vi "Project Names.vi"(8 "Error In":errorcluster, 11 "App In":refnum<vi>) -> (0 "Error Out":errorcluster, 2 "Project Names":string[](array[string]), 3 "App Out":refnum<vi>)   [LabVIEW 2017, in "Bookmark Manager.lvlib"]
uses:
  Bookmark Manager.lvlib
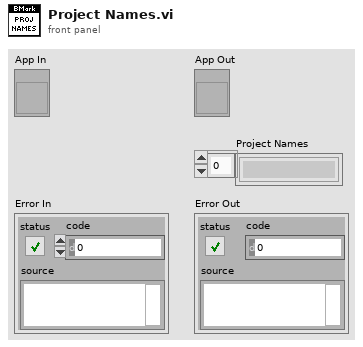
[diagram p1: front panel]
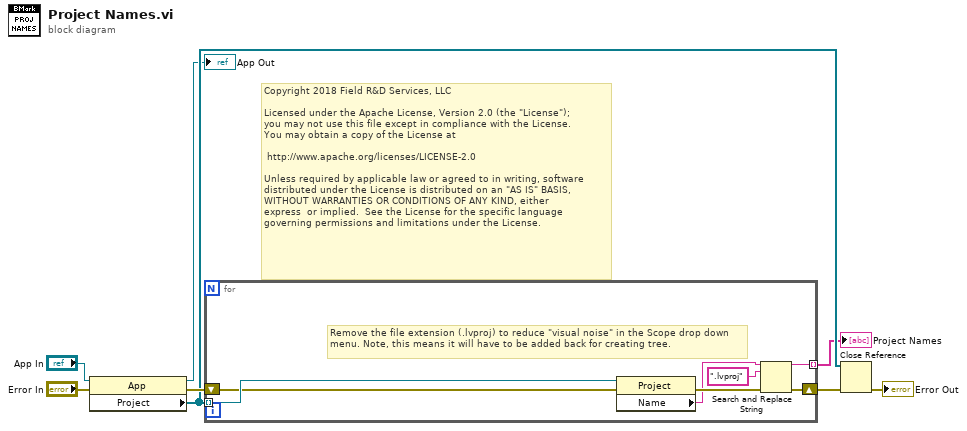
[diagram p0: block diagram]
diagram:
  # "Copyright 2018 Field R&D Services, LLC\n\nLicensed under the Apache License, Version 2.0 (the \"License\");\nyou may not use this file except in compliance with the License.\nYou may obtain a copy of the License at\n\n\thttp://www.apache.org/licenses/LICENSE-2.0\n\nUnless required by applicable law or agreed to in writing, software\ndistributed under the License is distributed on an \"AS IS\" BASIS,\nWITHOUT WARRANTIES OR CONDITIONS OF ANY KIND, either \nexpress  or implied.  See the License for the specific language \ngoverning permissions and limitations under the License."
  n1 = property class="App"(reference="App In", error in="Error In") -> (reference out=→"App Out":refnum<vi>, error out=w7:errorcluster, "Project"=w5:refnum<vi>[])
  n2 = for {
    shift-right: [w12] -> w6
    shift-left: w7 -> [w14]
    tunnel: w5 -> [w15] mode=indexing
    tunnel: [w9] -> w1 mode=indexing
    # "Remove the file extension (.lvproj) to reduce \"visual noise\" in the Scope drop down menu. Note, this means it will have to be added back for creating tree."
    n3 = property class="Project"(reference=w15, error in=w14) -> (error out=w13:errorcluster, "Name"=w11:string)  [unwired: 1 out]
    n4 = Search and Replace String(input string=w11, search string=".lvproj", error in=w13) -> (result string=w9:string, error out=w12:errorcluster)  [unwired: 5 in, 2 out]
  }
  "Project Names" <- w1
  n5 = Close Reference(reference=w5, error in (no error)=w6) -> (error out=→"Error Out":errorcluster)
